vi "functions_of_arrays.vi"() -> ()   [LabVIEW 2019]
panel:
  out "deleted portion":dbl[][](array[numeric])
  out "array w/ subset deleted":dbl[][](array[numeric])
  out "insert into array O/P":dbl[][](array[numeric])
  out "replace array subset O/P":dbl[][](array[numeric])
  in  "Sub array":dbl[][](array[numeric])
  out "element":dbl
  out "size  of array function":i32[](array[numeric])
  in  "input array":dbl[][](array[numeric])
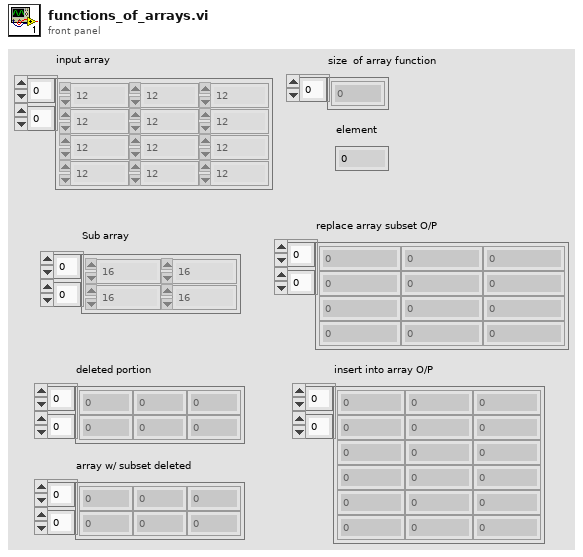
[diagram p1: front panel]
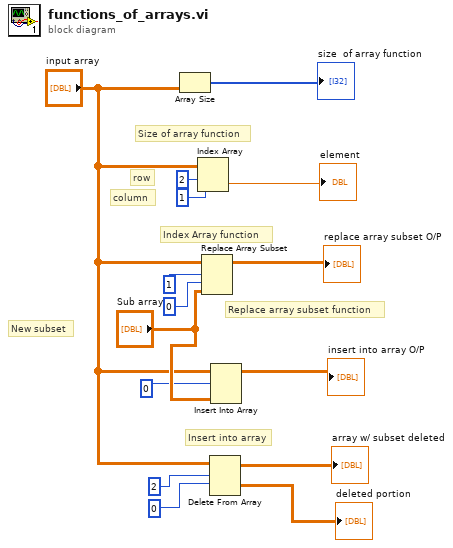
[diagram p0: block diagram]
diagram:
  # "Insert into array"
  # "New subset"
  # "Replace array subset function"
  # "column"
  # "row"
  # "Index Array function"
  # "Size of array function"
  n1 = Array Size(array="input array") -> (size(s)=→"size  of array function":i32[])
  n2 = Index Array(array="input array", index (row)=2, index (col)=1 ("disabled index (col)")) -> (element=→"element":dbl)
  n3 = Replace Array Subset(array="input array", new element="Sub array", index (row)=1, index (col)=0) -> (→"replace array subset O/P":dbl[][])
  n4 = Delete From Array(array="input array", length=2, index (row)=0) -> (deleted portion=→"deleted portion":dbl[][], array with subset deleted=→"array w/ subset deleted":dbl[][])  [unwired: 1 in]
  n5 = Insert Into Array(array="input array", index (row)=0, new element="Sub array") -> (→"insert into array O/P":dbl[][])  [unwired: 1 in]
